vi "Mayusculas (2).vi"(11 "Palabra":string) -> (1 "Boolean":bool, 2 "Numeric":u8, 3 "string":string)   [LabVIEW 2020]
doc: "Darlin y Miller: Subvi que detecta letras mayusculas por medio de la Tabla Ascii"
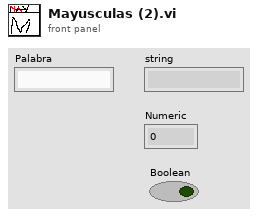
[diagram p1: front panel]
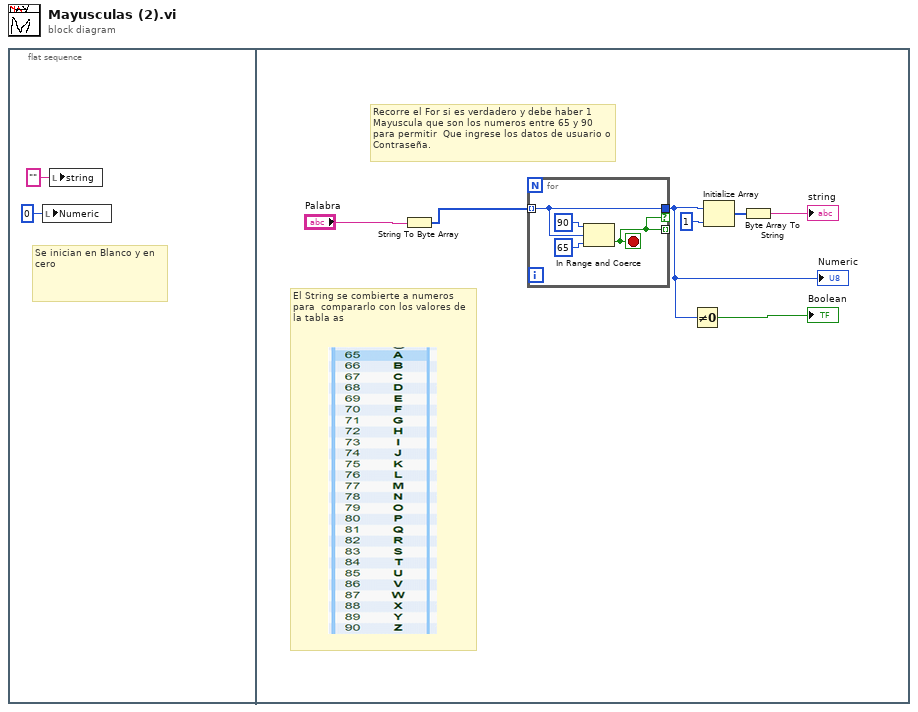
[diagram p0: block diagram]
diagram:
  n1 = flat-sequence {
    frame #0 {
      # "Se inician en Blanco y en cero"
      n2 = local write "Numeric"(u8 0 ("Numeric")) -> ()
      n3 = local write "string"("" ("string")) -> ()
    }
    frame #1 {
      # "Recorre el For si es verdadero y debe haber 1 Mayuscula que son los numeros entre 65 y 90 para permitir  Que ingrese los datos de usuario o Contraseña."
      # "El String se combierte a numeros para  compararlo con los valores de la tabla as"
      n4 = String To Byte Array(string="Palabra") -> (unsigned byte array=w3:u8[])
      n5 = for {
        tunnel: w3 -> [w10] mode=indexing
        tunnel: [w10] -> w8 if=w11
        tunnel: [w11] -> _ mode=indexing
        stop <- w11 stop-if-true
        n6 = In Range and Coerce(upper limit=u8 90, x=w10, lower limit=u8 65) -> (In Range?=w11:bool)  [unwired: 1 out]
      }
      "Numeric" <- w8
      n7 = Not Equal To 0?(x=w8) -> (x != 0?=→"Boolean":bool)
      n8 = Initialize Array "Initialize Array"(w8, 1 ("dimension size")) -> (w7:u8[])
      n9 = Byte Array To String(unsigned byte array=w7) -> (string=→"string":string)
    }
  }
